vi "RedisTab-DeviceCMD.vi"(7 "DeviceData":T2) -> ()   [LabVIEW 2020]
uses:
  MainFrame/Queue/queue.ctl
panel:
  out "RedisTabCondition2Update":string
  out "RedisTabName2Update":string
  out "Array":T1(array[cluster])
  out "Name":string
  out "CMD":T3
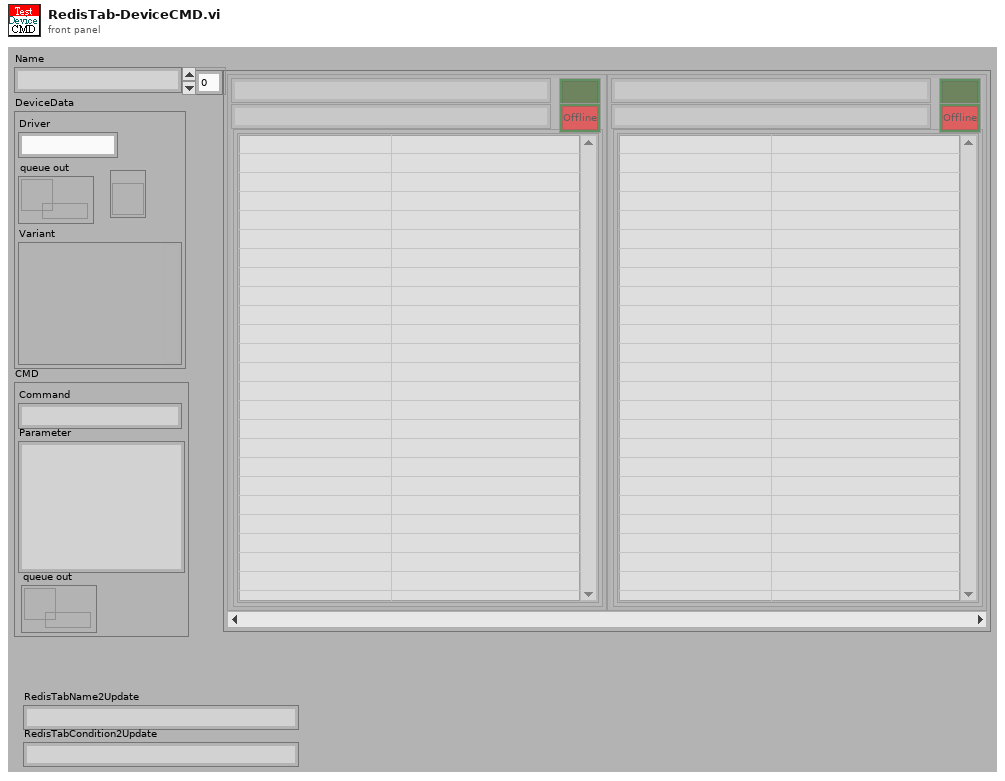
[diagram p1: front panel]
types:
  T1 = cluster{"CronTabName":string, "Condition":string, cluster{"Script":string[][]}, "Enable?":bool, "Link?":bool}[]
  T2 = cluster{"Driver":string, "queue out":refnum<queue>, refnum<vi>, "Variant":variant}
  T3 = cluster{"Command":string, "Parameter":string, "queue out":refnum<queue>}
  T4 = typedef "queue.ctl" = enum16{"RT queue Init", "Module queue Init", "Recieve queue Init", "CMD EXE queue Init", "Get queue", "release all queue"}
  T5 = cluster{"RedisTabName":string, "Condition":string, "Script":cluster{"Script":string[][]}, "Enable?":bool, "Link":bool}
  T6 = enum16{"Init", "Add", "Enable", "Disable", "Get", "UpdateVI"}
  T7 = enum16{"Get", "Init", "Set", "Delete", "GetElement", "Inc", "Dec", "ReName", "Copy"}
  T8 = enum16{"Init", "Add", "Enable", "Disable", "Get"}
  T9 = cluster{"RedisTabName":string, "Condition":string, "Script":cluster{"Script":string[][]}, "Enable?":bool, "Link":bool}[]
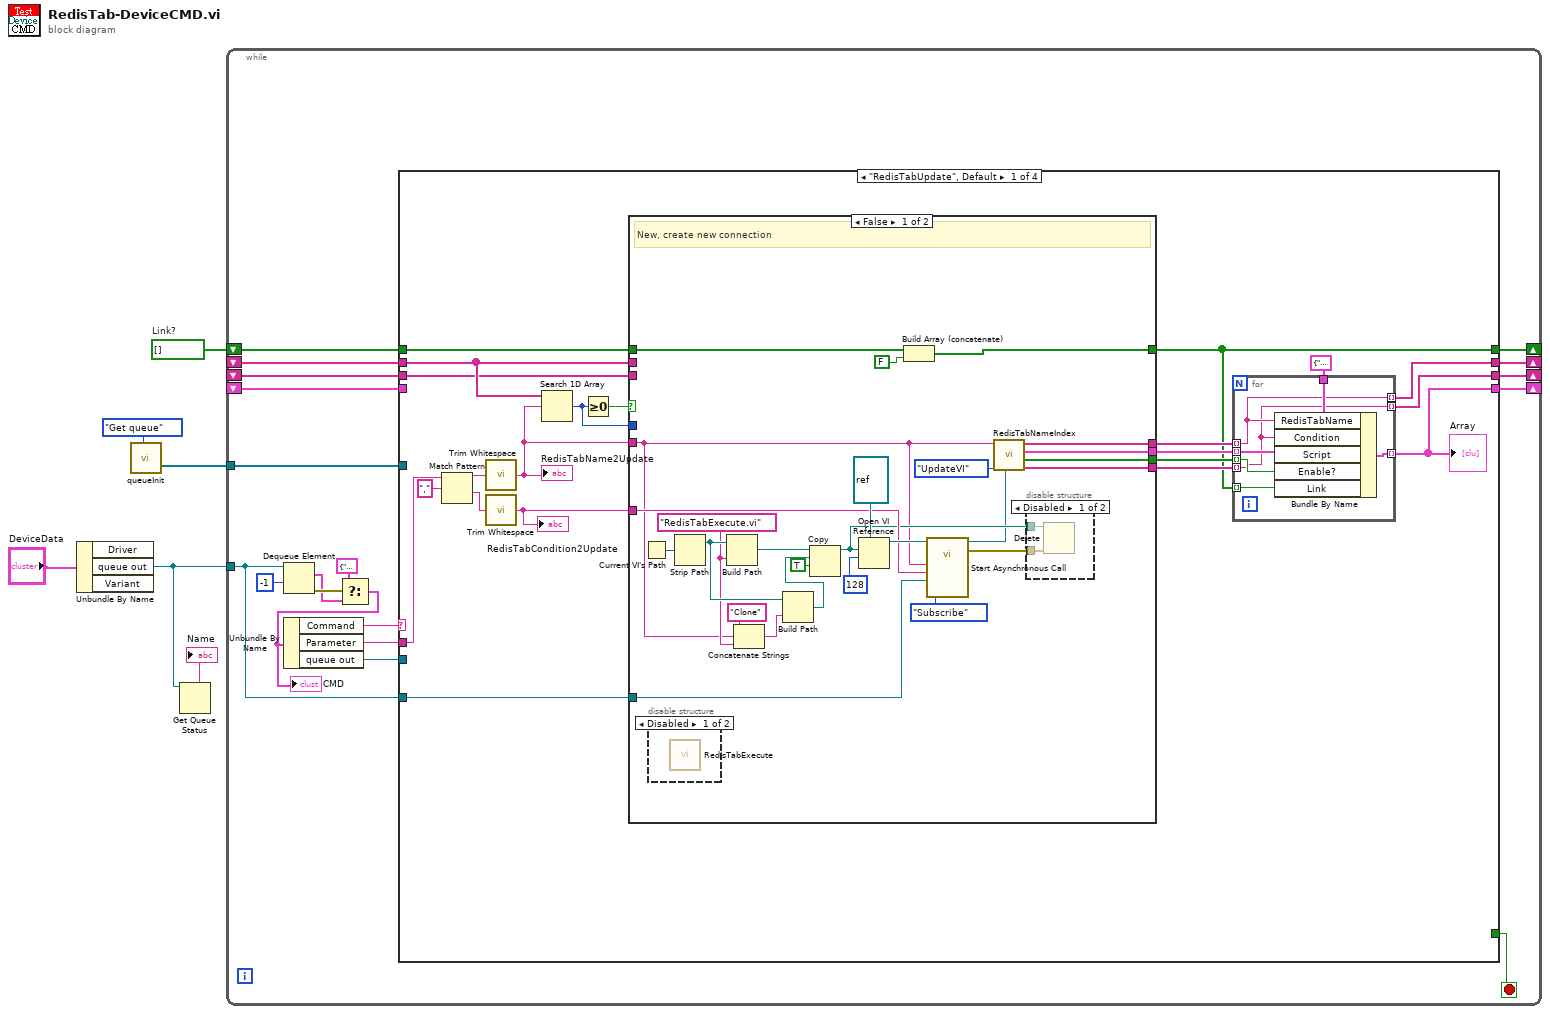
[diagram p0: block diagram]
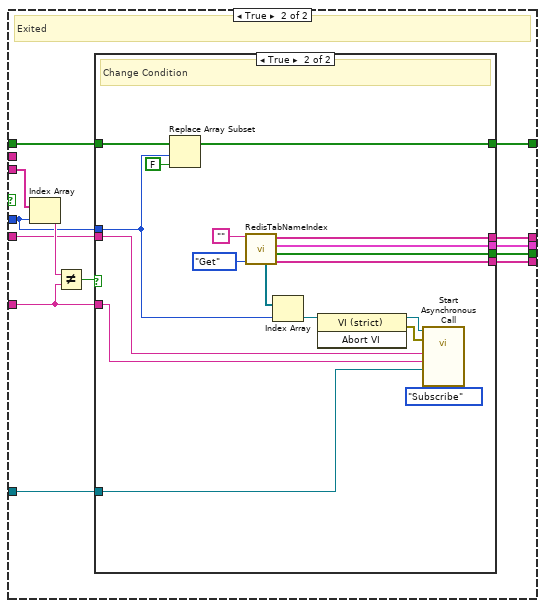
[diagram p4: hidden frame]
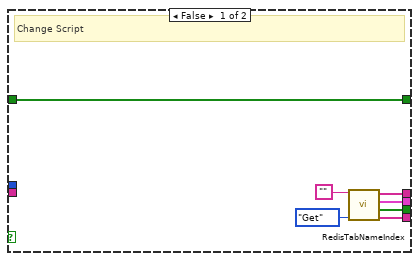
[diagram p5: hidden frame]
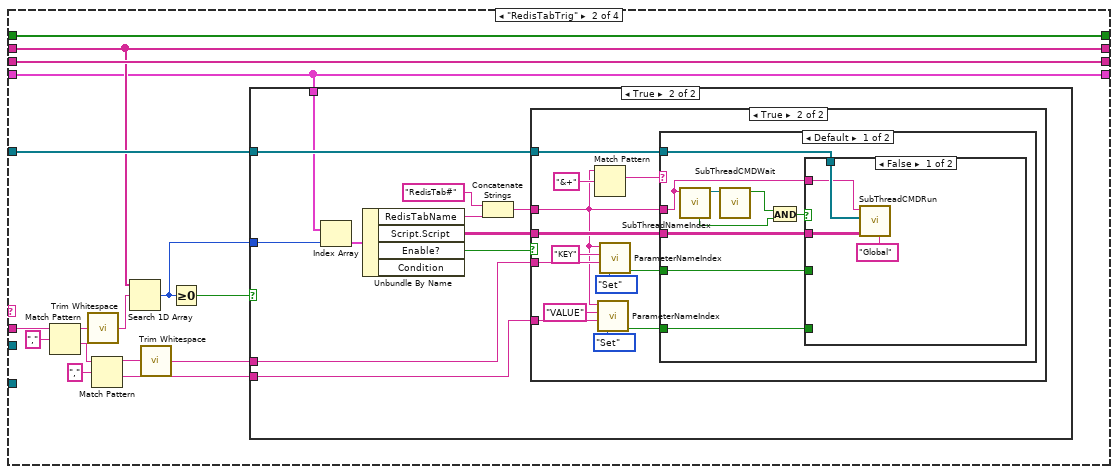
[diagram p6: hidden frame]
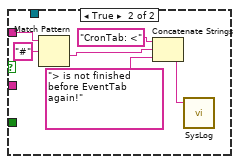
[diagram p9: hidden frame]
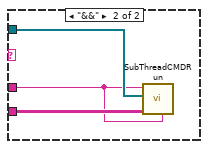
[diagram p10: hidden frame]
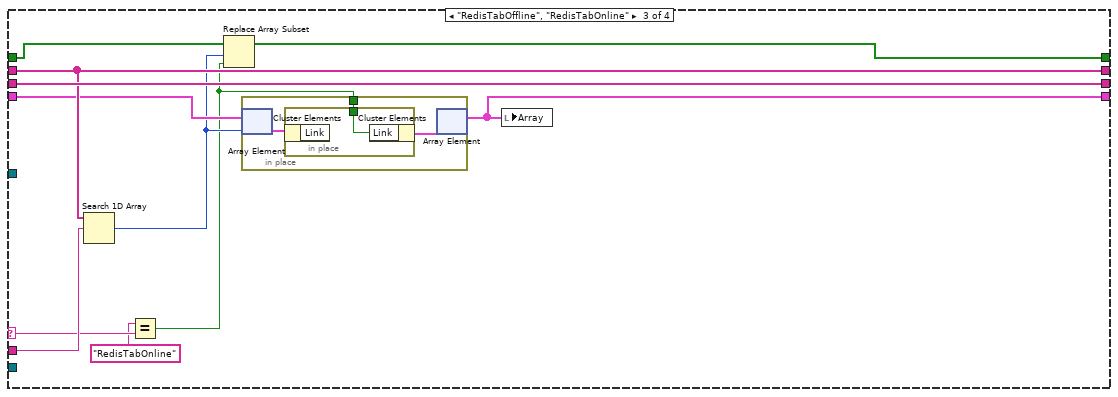
[diagram p11: hidden frame]
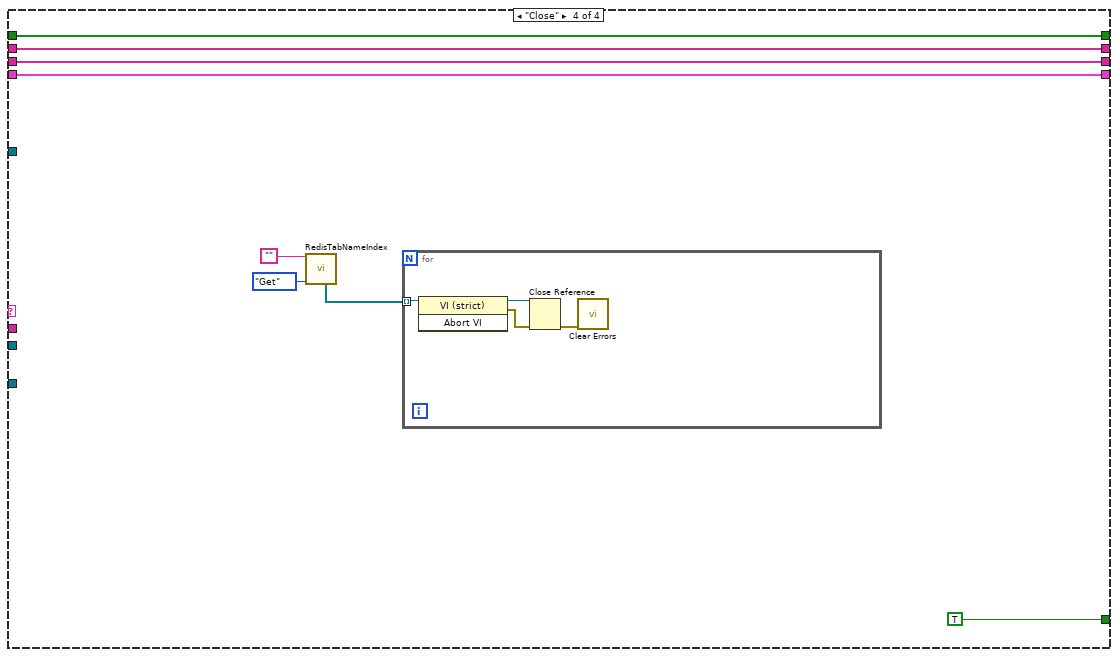
[diagram p12: hidden frame]
diagram:
  w1 = bool[] []  # Link?
  n1 = Unbundle By Name("DeviceData") -> ("queue out"=w2:refnum<queue>)  [unwired: 2 out]
  n2 = call "queueInit.vi"("CMD"=queue."Get queue") -> ("CMD EXE thread queue"=w3:refnum<queue>[])  [unwired: 14 in, 4 out]
  n3 = Get Queue Status(queue=w2) -> (queue name=→"Name":string)  [unwired: 2 in, 7 out]
  n4 = while {
    tunnel: w2 -> [w9]
    shift-right: [w16] -> _
    shift-left: _ -> [w15]
    tunnel: w3 -> [w14]
    shift-right: [w13] -> _
    shift-left: _ -> [w11]
    shift-right: [w12] -> _
    shift-left: _ -> [w10]
    shift-right: [w7] -> _
    shift-left: w1 -> [w8]
    stop <- w22 stop-if-true
    n5 = Dequeue Element(queue=w9, timeout in ms (-1)=-1) -> (element=w19:T3, error out=w20:errorcluster)  [unwired: 1 in, 2 out]
    n6 = Select(t=T3 {"Command"="Close", "Parameter"="", "queue out"=refnum}, s=w20, f=w19) -> (s? t:f=w18:T3)
    "CMD" <- w18
    n7 = Unbundle By Name(w18) -> ("Command"=w25:string, "Parameter"=w24:string, "queue out"=w23:refnum<queue>)
    n8 = case shown="\"RedisTabUpdate\", Default" w25 {
      selector: w25 -> [_ _ w184 _]
      tunnel: w24 -> [w44 w134 w190 _]
      tunnel: w23 -> [_ _ _ _]
      tunnel: [_ _ _ TRUE] -> w22
      tunnel: [w46 w123 w185 w203] -> w16
      tunnel: w15 -> [_ w123 w187 w203]
      tunnel: w14 -> [_ w135 _ _]
      tunnel: [w42 w124 w191 w202] -> w13
      tunnel: [w41 w131 w192 w201] -> w12
      tunnel: w11 -> [w35 w124 w191 w202]
      tunnel: w10 -> [w34 w131 w192 w201]
      tunnel: w9 -> [w32 _ _ _]
      tunnel: w8 -> [w27 w120 w189 w197]
      tunnel: [w26 w120 w188 w197] -> w7
      frame "RedisTabUpdate", Default {
        n9 = Match Pattern(string=w44, regular expression=",") -> (before substring=w40:string, after substring=w39:string)  [unwired: 1 in, 2 out]
        n10 = call <vilib>:"Trim Whitespace.vi"("string"=w40) -> ("trimmed string"=w37:string)  [unwired: 1 in]
        "RedisTabName2Update" <- w37
        n11 = call <vilib>:"Trim Whitespace.vi"("string"=w39) -> ("trimmed string"=w33:string)  [unwired: 1 in]
        "RedisTabCondition2Update" <- w33
        n12 = Search 1D Array(1D array=w35, element=w37) -> (index of element=w36:i32)  [unwired: 1 in]
        n13 = Greater Or Equal To 0?(x=w36) -> (x >= 0?=w38:bool)
        n14 = case shown="False" w38 {
          tunnel: w37 -> [w57 w79]
          tunnel: w36 -> [_ w84]
          tunnel: w35 -> [_ _]
          tunnel: w34 -> [_ w87]
          tunnel: w33 -> [w69 w78]
          tunnel: w32 -> [w68 w77]
          tunnel: [w53 w83] -> w31
          tunnel: [w52 w82] -> w30
          tunnel: [w51 w81] -> w29
          tunnel: [w50 w80] -> w28
          tunnel: w27 -> [w49 w76]
          tunnel: [w47 w75] -> w26
          frame False {
            w63 = "RedisTabExecute.vi"
            # "New, create new connection"
            n15 = Current VI's Path() -> (path=w71:path)
            n16 = disable-structure shown="Disabled" {
              frame Disabled {
                n17 = call "RedisTabExecute.vi"() -> ()  [unwired: 12 in]
              }
              frame Enabled {
              }
            }
            n18 = Strip Path(path=w71) -> (stripped path=w64:path)  [unwired: 1 out]
            n19 = Build Path(base path=w64, name or relative path=w63) -> (appended path=w66:path)
            n20 = Concatenate Strings("Clone" ("string"), w57, w63) -> (w61:string)
            n21 = Build Path(base path=w64, name or relative path=w61) -> (appended path=w60:path)
            n22 = Copy(9:TRUE ("overwrite (F)"), 10:w60, 11:w66) -> (3:w58:path)  [unwired: 2 in, 2 out]
            n23 = Open VI Reference(type specifier VI Refnum (for type only)=refnum<vi> refnum, vi path=w58, options=128) -> (vi reference=w70:refnum<vi>)  [unwired: 3 in, 1 out]
            n24 = Build Array (concatenate)(w49, FALSE) -> (w47:bool[])
            n25 = call-by-ref "Start Asynchronous Call"(reference=w70, "Type"=enum16{"Subscribe", "LPop", "Stream"}."Subscribe", "RedisTabQueue"=w68, "RedisTabCondition"=w69, "RedisTabName"=w57) -> (reference out=w55:refnum<vi>, error out=w59:errorcluster)  [unwired: 9 in]
            n26 = call "RedisTabNameIndex.vi"("RedisTabExecute"=w55, "OP"=T6."UpdateVI", "RedisTabName"=w57) -> ("RedisTableConditionS"=w50:string[], "Enable?S"=w51:bool[], "Scripts"=w52:cluster{"Script":string[][]}[], "RedisTabNameS"=w53:string[])  [unwired: 4 in, 1 out]
            n27 = disable-structure shown="Disabled" {
              disable-tunnel: w59 -> [w74 _]
              disable-tunnel: w58 -> [w73 _]
              frame Disabled {
                n28 = Delete(path (use dialog)=w73, error in=w74) -> ()  [unwired: 3 in, 3 out]
              }
              frame Enabled {
              }
            }
          }
          frame True {
            # "Exited"
            n29 = Index Array(array=w87, index=w84) -> (element=w86:string)
            n30 = Not Equal?(x=w86, y=w78) -> (x != y?=w85:bool)
            n31 = case shown="True" w85 {
              tunnel: w84 -> [_ w98]
              tunnel: [w92 w103] -> w83
              tunnel: [w91 w102] -> w82
              tunnel: [w90 w101] -> w81
              tunnel: [w89 w100] -> w80
              tunnel: w79 -> [_ w106]
              tunnel: w78 -> [_ w105]
              tunnel: w77 -> [_ w104]
              tunnel: w76 -> [w88 w99]
              tunnel: [w88 w96] -> w75
              frame False {
                # "Change Script"
                n32 = call "RedisTabNameIndex.vi"("OP"=T6."Get", "RedisTabName"="") -> ("RedisTableConditionS"=w89:string[], "Enable?S"=w90:bool[], "Scripts"=w91:cluster{"Script":string[][]}[], "RedisTabNameS"=w92:string[])  [unwired: 5 in, 1 out]
              }
              frame True {
                # "Change Condition"
                n33 = Replace Array Subset(array=w99, new element=FALSE ("new element/subarray"), index=w98) -> (w96:bool[])
                n34 = call "RedisTabNameIndex.vi"("OP"=T6."Get", "RedisTabName"="") -> ("RedisTableConditionS"=w100:string[], "Enable?S"=w101:bool[], "Scripts"=w102:cluster{"Script":string[][]}[], "RedisTabNameS"=w103:string[], "RedisTabExecuteS"=w95:refnum<vi>[])  [unwired: 5 in]
                n35 = Index Array(array=w95, index=w98) -> (element=w110:refnum<vi>)
                n36 = invoke class="VI (strict)" method="Abort VI"(reference=w110) -> (reference out=w109:refnum<vi>, error out=w107:errorcluster)  [unwired: 2 in, 1 out]
                n37 = call-by-ref "Start Asynchronous Call"(reference=w109, error in=w107, "Type"=enum16{"Subscribe", "LPop", "Stream"}."Subscribe", "RedisTabQueue"=w104, "RedisTabCondition"=w105, "RedisTabName"=w106) -> ()  [unwired: 8 in, 2 out]
              }
            }
          }
        }
        n38 = for {
          tunnel: w31 -> [w115] mode=indexing
          tunnel: w30 -> [w118] mode=indexing
          tunnel: w29 -> [w117] mode=indexing
          tunnel: w28 -> [w114] mode=indexing
          tunnel: [w116] -> w46 mode=indexing
          tunnel: T5 {"RedisTabName"="", "Condition"="", "Script"={"Script"=[]}, "Enable?"=TRUE, "Link"=FALSE} ("Cluster") -> [w119]
          tunnel: [w115] -> w42 mode=indexing
          tunnel: [w114] -> w41 mode=indexing
          tunnel: w26 -> [w113] mode=indexing
          n39 = Bundle By Name(cluster=w119, "RedisTabName"=w115, "Condition"=w114, "Script"=w118, "Enable?"=w117, "Link"=w113) -> (w116:T5)
        }
        "Array" <- w46
      }
      frame "RedisTabTrig" {
        n40 = Match Pattern(string=w134, regular expression=",") -> (before substring=w132:string, after substring=w129:string)  [unwired: 1 in, 2 out]
        n41 = call <vilib>:"Trim Whitespace.vi"("string"=w132) -> ("trimmed string"=w125:string)  [unwired: 1 in]
        n42 = Match Pattern(string=w129, regular expression=",") -> (before substring=w128:string, after substring=w126:string)  [unwired: 1 in, 2 out]
        n43 = Search 1D Array(1D array=w124, element=w125) -> (index of element=w122:i32)  [unwired: 1 in]
        n44 = call <vilib>:"Trim Whitespace.vi"("string"=w128) -> ("trimmed string"=w127:string)  [unwired: 1 in]
        n45 = Greater Or Equal To 0?(x=w122) -> (x >= 0?=w121:bool)
        n46 = case shown="True" w121 {
          tunnel: w135 -> [_ w146]
          tunnel: w127 -> [_ w141]
          tunnel: w126 -> [_ w140]
          tunnel: w123 -> [_ w139]
          tunnel: w122 -> [_ w138]
          frame False {
          }
          frame True {
            n47 = Index Array(array=w139, index=w138) -> (element=w137:T5)
            n48 = Unbundle By Name(w137) -> ("RedisTabName"=w145:string, "Script.Script"=w142:string[][], "Enable?"=w136:bool)  [unwired: 1 out]
            n49 = Concatenate Strings("RedisTab#" ("string"), w145) -> (w143:string)
            n50 = case shown="True" w136 {
              tunnel: w143 -> [_ w149]
              tunnel: w146 -> [_ w159]
              tunnel: w142 -> [_ w158]
              tunnel: w141 -> [_ w155]
              tunnel: w140 -> [_ w147]
              frame False {
              }
              frame True {
                n51 = Match Pattern(string=w149, regular expression="&+") -> (match substring=w148:string)  [unwired: 1 in, 3 out]
                n52 = call "ParameterNameIndex.vi"("OP"=T7."Set", "Value"=w147, "Key"="VALUE", "VariableSection"=w149) -> ("Find?"=w152:bool)  [unwired: 1 in, 6 out]
                n53 = call "ParameterNameIndex.vi"("OP"=T7."Set", "Value"=w155, "Key"="KEY", "VariableSection"=w149) -> ("Find?"=w156:bool)  [unwired: 1 in, 6 out]
                n54 = case shown="Default" w148 {
                  tunnel: w159 -> [w168 w180]
                  tunnel: w158 -> [w167 w181]
                  tunnel: w156 -> [w162 _]
                  tunnel: w152 -> [w161 _]
                  tunnel: w149 -> [w160 w179]
                  frame Default {
                    n55 = call "SubThreadNameIndex.vi"("SubThreadName"=w160) -> ("vi reference"=w166:refnum<vi>, "Find?"=w164:bool)  [unwired: 7 in, 2 out]
                    n56 = call "SubThreadCMDWait.vi"("vi reference"=w166) -> ("Run?"=w165:bool)  [unwired: 10 in]
                    n57 = And(x=w165, y=w164) -> (x .and. y?=w163:bool)
                    n58 = case shown="False" w163 {
                      tunnel: w168 -> [w172 _]
                      tunnel: w167 -> [w171 _]
                      tunnel: w160 -> [w170 w175]
                      tunnel: w162 -> [_ _]
                      tunnel: w161 -> [_ _]
                      frame False {
                        n59 = call "SubThreadCMDRun.vi"("ID#CallBack"="Global", "Command"=w171, "Threads"=w172, "SubThreadName"=w170) -> ()  [unwired: 7 in, 1 out]
                      }
                      frame True {
                        n60 = Match Pattern(string=w175, regular expression="#") -> (after substring=w173:string)  [unwired: 1 in, 3 out]
                        n61 = Concatenate Strings("CronTab: <", w173, "> is not finished before EventTab again!" ("string")) -> (w176:string)
                        n62 = call "SysLog.vi"("Mssage"=w176) -> ()  [unwired: 5 in]
                      }
                    }
                  }
                  frame "&&" {
                    n63 = call "SubThreadCMDRun.vi"("ID#CallBack"=w179, "Command"=w181, "Threads"=w180, "SubThreadName"=w179) -> ()  [unwired: 7 in, 1 out]
                  }
                }
              }
            }
          }
        }
      }
      frame "RedisTabOffline", "RedisTabOnline" {
        n64 = Search 1D Array(1D array=w191, element=w190) -> (index of element=w186:i32)  [unwired: 1 in]
        n65 = Equal?(x="RedisTabOnline", y=w184) -> (x = y?=w182:bool)
        n66 = Replace Array Subset(array=w189, new element=w182, index=w186) -> (w188:bool[])
        n67 = in-place {
          in-place-border: w182 -> [w194]
          n68 = in-place-array #1(w187, w186) -> (w195:T5)
          n69 = in-place {
            in-place-border: w194 -> [w196]
            n70 = in-place-cluster #2(w195) -> ()  [unwired: 1 out]
            n71 = in-place-cluster #2("Link"=w196) -> (w193:T5)
          }
          n72 = in-place-array #1(w193) -> (w185:T9)  [unwired: 1 out]
        }
        n73 = local write "Array"(w185) -> ()
      }
      frame "Close" {
        n74 = call "RedisTabNameIndex.vi"("OP"=T8."Get", "RedisTabName"="") -> ("RedisTabExecuteS"=w198:refnum<vi>[])  [unwired: 5 in, 4 out]
        n75 = for {
          tunnel: w198 -> [w207] mode=indexing
          n76 = invoke class="VI (strict)" method="Abort VI"(reference=w207) -> (reference out=w206:refnum<vi>, error out=w205:errorcluster)  [unwired: 2 in, 1 out]
          n77 = Close Reference(reference=w206, error in (no error)=w205) -> (error out=w208:errorcluster)
          n78 = call <vilib>:"Clear Errors.vi"("error in (no error)"=w208) -> ()  [unwired: 5 in, 2 out]
        }
      }
    }
  }
